vi "Report Auton Action.vi"(8 "error in":errorcluster, 9 "Aborted?":bool, 10 "Name":string, 11 "Auton Monitor":T1) -> (0 "error out":errorcluster)   [LabVIEW 2016, in "Auton Mode Base.lvclass"]
uses:
  Auton Mode Base.lvclass
  Auton Action Monitor Type.ctl
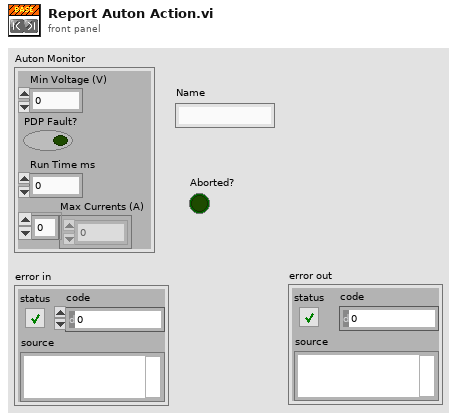
[diagram p1: front panel]
types:
  T1 = typedef "Auton Mode Base.lvclass/Auton Action Monitor Type.ctl" = cluster{"Min Voltage (V)":dbl, "PDP Fault?":bool, "Run Time ms":u32, "Max Currents (A)":dbl[]}
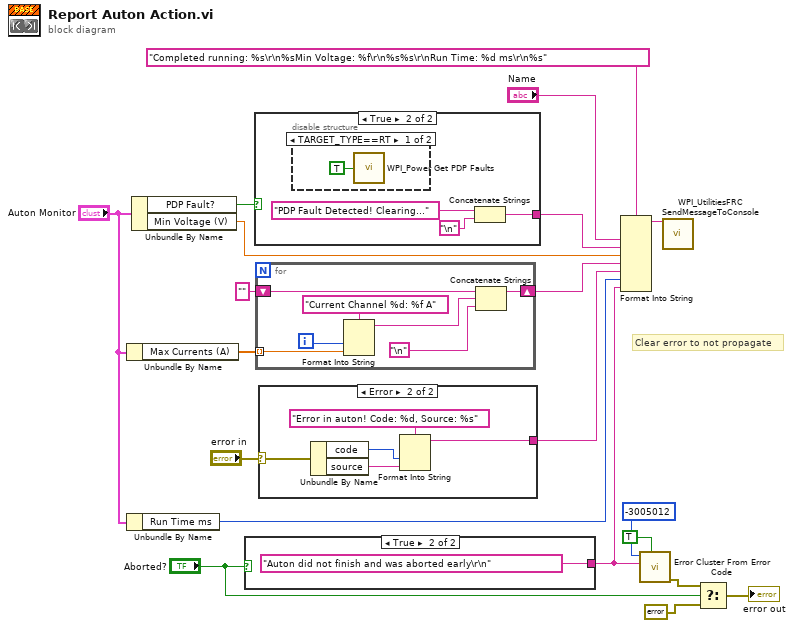
[diagram p0: block diagram]
diagram:
  # "Clear error to not propagate"
  n1 = Unbundle By Name("Auton Monitor") -> ("Max Currents (A)"=w19:dbl[])
  n2 = Unbundle By Name("Auton Monitor") -> ("Run Time ms"=w8:u32)
  n3 = Unbundle By Name("Auton Monitor") -> ("PDP Fault?"=w17:bool, "Min Voltage (V)"=w14:dbl)
  n4 = case shown="True" "Aborted?" {
    tunnel: [_ "Auton did not finish and was aborted early\r\n" ("format string")] -> w4
    frame False {
    }
    frame True {
    }
  }
  n5 = case shown="True" w17 {
    tunnel: [_ w22] -> w16
    frame False {
    }
    frame True {
      n6 = disable-structure shown="TARGET_TYPE==RT" {
        frame condition #0 (active) {
          n7 = call <vilib>:"WPI_Power Get PDP Faults.vi"("Clear Sticky Faults"=TRUE) -> ()  [unwired: 10 in, 5 out]
        }
        frame condition #1 {
        }
      }
      n8 = Concatenate Strings("PDP Fault Detected! Clearing..." ("format string"), "\n") -> (w22:string)
    }
  }
  n9 = for {
    tunnel: w19 -> [w32] mode=indexing
    shift-right: [w28] -> w13
    shift-left: "" -> [w29]
    i -> [w31]
    n10 = Format Into String(format string="Current Channel %d: %f A", w31, w32) -> (resulting string=w27:string)  [unwired: 2 in, 1 out]
    n11 = Concatenate Strings(w29, w27, "\n") -> (w28:string)
  }
  n12 = case shown="Error" "error in" {
    selector: "error in" -> [_ w37]
    tunnel: [_ w33] -> w12
    frame No Error {
    }
    frame Error {
      n13 = Unbundle By Name(w37) -> ("code"=w36:i32, "source"=w35:string)
      n14 = Format Into String(format string="Error in auton! Code: %d, Source: %s", w36, w35) -> (resulting string=w33:string)  [unwired: 2 in, 1 out]
    }
  }
  n15 = Format Into String(format string="Completed running: %s\r\n%sMin Voltage: %f\r\n%s%s\r\nRun Time: %d ms\r\n%s", "Name", w16, w14, w13, w12, w8, w4) -> (resulting string=w11:string)  [unwired: 2 in, 1 out]
  n16 = call <vilib>:"Error Cluster From Error Code.vi"("show call chain? (False)"=TRUE, "error message (\"\")"=w4, "error code (0)"=-3005012) -> ("error out"=w3:errorcluster)  [unwired: 6 in]
  n17 = call <vilib>:"WPI_UtilitiesFRC SendMessageToConsole.vi"("Message"=w11) -> ()  [unwired: 14 in, 1 out]
  n18 = Select(t=w3, s="Aborted?", f=errorcluster {"status"=FALSE, "code"=0, "source"=""} ("error out")) -> (s? t:f=→"error out":errorcluster)
